vi "Get Control Reference by Label (1D STR).vi"(8 "error in (no error)":errorcluster, 10 "Control Names":string[](array[string]), 11 "Control Ref Map":map{string, refnum<vi>}(c390)) -> (0 "error out":errorcluster, 2 "Found?":bool, 3 "Control Refs":refnum<vi>[](array[refnum]))   [LabVIEW 2020, in "MacroAssert.lvlib"]
doc: "Gets the references of <B>Control Names</B> from <B>Control Ref Map</B>."
uses:
  MacroAssert.lvlib
  <vilib>/Utility/error.llb/Error Cluster From Error Code.vi
  SubVIs/Custom Errors/Custom Errors.lvlib
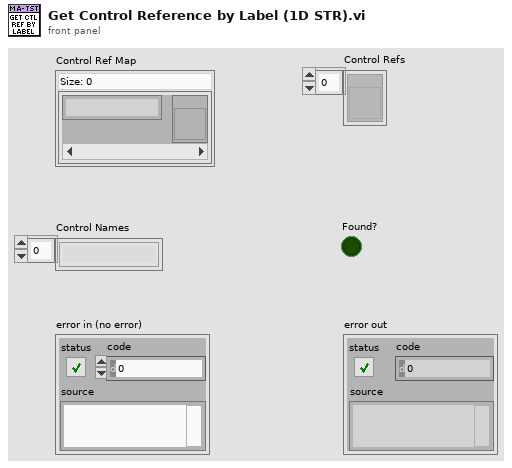
[diagram p1: front panel]
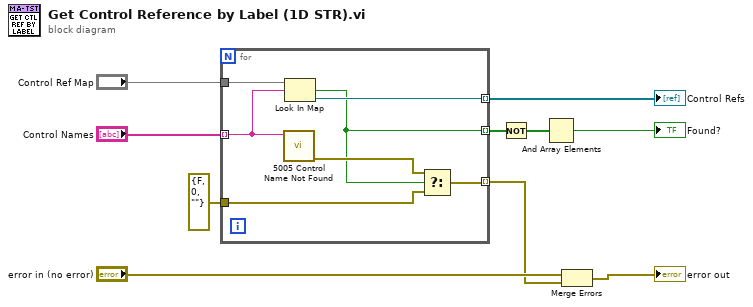
[diagram p0: block diagram]
diagram:
  n1 = for {
    tunnel: "Control Ref Map" -> [w17]
    tunnel: [w15] -> w7 mode=indexing
    tunnel: "Control Names" -> [w14] mode=indexing
    tunnel: [w13] -> w5 mode=indexing
    tunnel: [w12] -> w4 mode=indexing
    tunnel: errorcluster {"status"=FALSE, "code"=0, "source"=""} ("error in (no error)") -> [w11]
    n2 = call "5005 Control Name Not Found.vi"("Control Name"=w14) -> ("error out"=w16:errorcluster)  [unwired: 10 in]
    n3 = Look In Map(map=w17, key=w14) -> (key not found?=w12:bool, value=w13:refnum<vi>)  [unwired: 1 in]
    n4 = Select(t=w16, s=w12, f=w11) -> (s? t:f=w15:errorcluster)
  }
  "Control Refs" <- w5
  n5 = Not(x=w4) -> (.not. x?=w3:bool[])
  n6 = And Array Elements(Boolean array=w3) -> (logical AND=→"Found?":bool)
  n7 = Merge Errors("error in (no error)", w7) -> (→"error out":errorcluster)
